vi "get_voltage.vi"(8 "Error in":errorcluster, 10 "Bytes of voltage":u8[](array[numeric])) -> (0 "Error out":errorcluster, 2 "Voltage [V]":dbl)   [LabVIEW 2020]
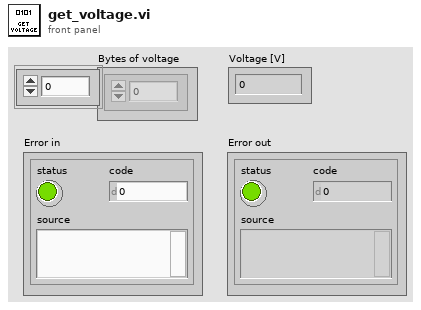
[diagram p1: front panel]
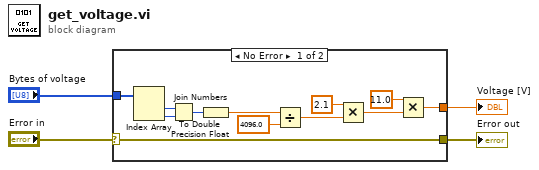
[diagram p0: block diagram]
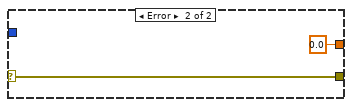
[diagram p2: hidden frame]
diagram:
  n1 = case shown="No Error" "Error in" {
    selector: "Error in" -> [w5 w18]
    tunnel: "Bytes of voltage" -> [w16 _]
    tunnel: [w15 0.0] -> w3
    tunnel: [w5 w18] -> w1
    frame No Error {
      n2 = Index Array(array=w16) -> (element #1=w12:u8, element #2=w13:u8)  [unwired: 2 in]
      n3 = Join Numbers(hi=w12, lo=w13) -> ((hi.lo)=w14:u16)
      n4 = To Double Precision Float(number=w14) -> (double precision float=w6:dbl)
      n5 = Divide(x=w6, y=4096.0 ("time informations.dt[s]")) -> (x/y=w8:dbl)
      n6 = Multiply(x=2.1 ("time informations.dt[s]"), y=w8) -> (x*y=w11:dbl)
      n7 = Multiply(x=11.0 ("time informations.dt[s]"), y=w11) -> (x*y=w15:dbl)
    }
    frame Error {
    }
  }
  "Voltage [V]" <- w3
  "Error out" <- w1
